vi "BCtr_acq.vi"(8 "error in (no error)":errorcluster, 11 "CtrCfg":T1 {"BaseAddrOut" format="%x"}) -> (0 "error out":errorcluster, 2 "Ack":bool, 3 "Values":u16[](array[numeric]) format="%x")   [LabVIEW 2016]
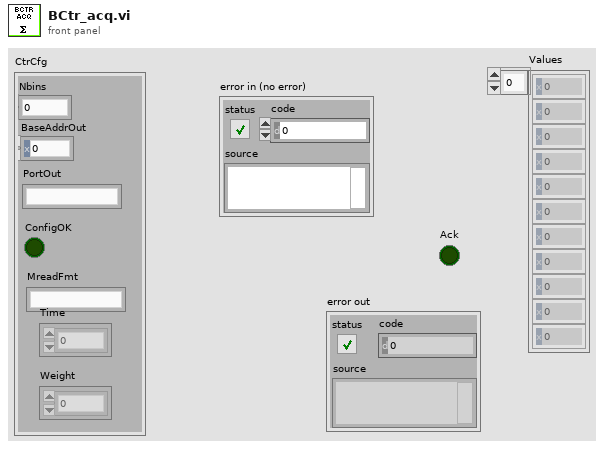
[diagram p1: front panel]
types:
  T1 = cluster{"Nbins":u16, "BaseAddrOut":u16, "PortOut":string, "ConfigOK":bool, "MreadFmt":string, "Time":dbl[], "Weight":dbl[]}
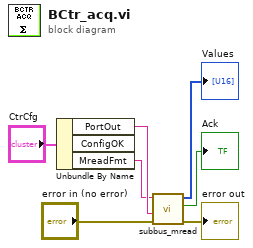
[diagram p0: block diagram]
diagram:
  n1 = Unbundle By Name("CtrCfg") -> ("PortOut"=w4:string, "MreadFmt"=w2:string)  [unwired: 1 out]
  n2 = call "subbus_mread.vi"("error in (no error)"="error in (no error)", "Port"=w4, "Cmd"=w2) -> ("error out"=→"error out":errorcluster, "Ack"=→"Ack":bool, "Values"=→"Values":u16[])  [unwired: 5 in, 1 out]
